vi "save_to_disk.vi"(1 "character string":string, 2 "Array":dbl[][](array[numeric]), 3 "File identifier":string) -> (0 "path":path)   [LabVIEW 2013]
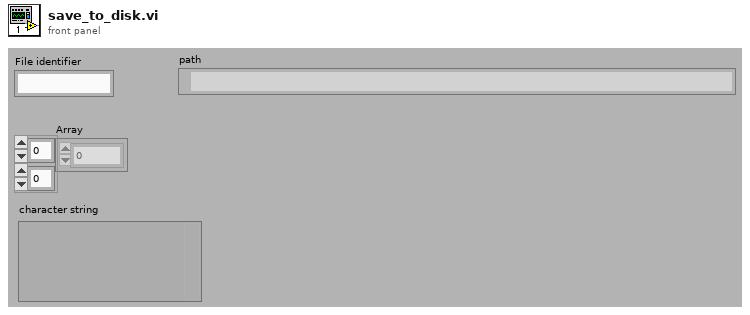
[diagram p1: front panel]
types:
  T1 = enum16{"open", "replace", "create", "open or create", "replace or create", "replace or create with confirmation"}
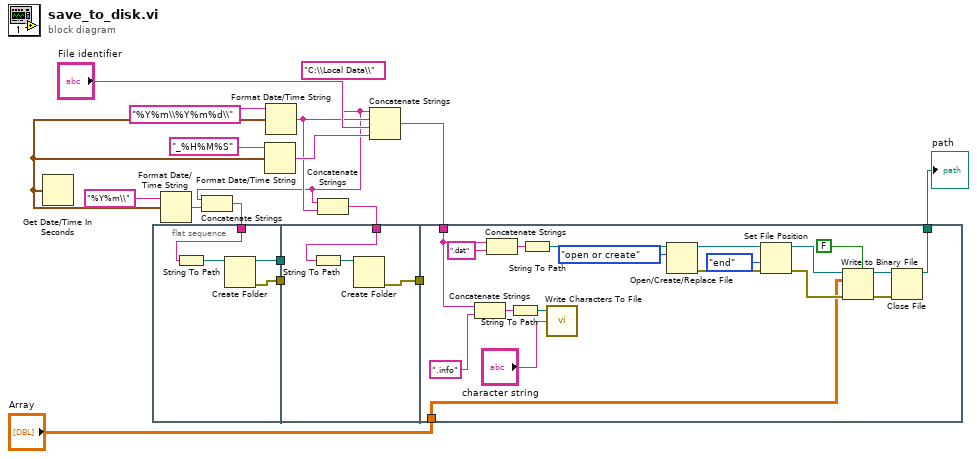
[diagram p0: block diagram]
diagram:
  w6 = "C:\\Local Data\\" ("string")
  n1 = Get Date/Time In Seconds() -> (seconds since 1Jan1904=w11:timestamp)
  n2 = flat-sequence {
    tunnel: [w21] -> w17
    tunnel: w4 -> [w20]
    tunnel: [w18] -> w1
    tunnel: w17 -> [_]
    tunnel: [w24] -> w16
    tunnel: w5 -> [w22]
    tunnel: w1 -> [_]
    tunnel: "Array" -> [w26]
    tunnel: w16 -> [_]
    tunnel: w3 -> [w40]
    tunnel: [w25] -> w2
    frame #0 {
      n3 = String To Path(string=w20) -> (path=w19:path)
      n4 = Create Folder(path (use dialog)=w19) -> (created path=w18:path, error out=w21:errorcluster)  [unwired: 2 in, 1 out]
    }
    frame #1 {
      n5 = String To Path(string=w22) -> (path=w23:path)
      n6 = Create Folder(path (use dialog)=w23) -> (error out=w24:errorcluster)  [unwired: 2 in, 2 out]
    }
    frame #2 {
      n7 = Concatenate Strings(w40, ".info" ("string")) -> (w38:string)
      n8 = Concatenate Strings(w40, ".dat" ("string")) -> (w43:string)
      n9 = String To Path(string=w38) -> (path=w39:path)
      n10 = String To Path(string=w43) -> (path=w28:path)
      n11 = call <vilib>:"Write Characters To File.vi"("character string"="character string", "file path (dialog if empty)"=w39) -> ()  [unwired: 3 in, 1 out]
      n12 = Open/Create/Replace File(file path (use dialog)=w28, operation (0:open)=T1."open or create") -> (refnum out=w35:refnum<file>, error out=w30:errorcluster)  [unwired: 4 in, 1 out]
      n13 = Set File Position(refnum=w35, from (0:start)=enum16{"start", "end", "current"}."end", error in=w30) -> (refnum out=w34:refnum<file>, error out=w31:errorcluster)  [unwired: 1 in]
      n14 = Write to Binary File(file (use dialog)=w34, data=w26, error in=w31, 5:FALSE ("prepend array or string size? (T)")) -> (refnum out=w32:refnum<file>, error out=w33:errorcluster)  [unwired: 2 in, 1 out]
      n15 = Close File(refnum=w32, error in=w33) -> (path=w25:path)  [unwired: 1 out]
    }
  }
  n16 = Format Date/Time String(time format string (%c)="%Y%m\\", seconds (now)=w11) -> (date/time string=w10:string)  [unwired: 1 in]
  n17 = Concatenate Strings(w6, w10) -> (w4:string)
  n18 = Format Date/Time String(time format string (%c)="_%H%M%S", seconds (now)=w11) -> (date/time string=w13:string)  [unwired: 1 in]
  n19 = Format Date/Time String(time format string (%c)="%Y%m\\%Y%m%d\\", seconds (now)=w11) -> (date/time string=w9:string)  [unwired: 1 in]
  n20 = Concatenate Strings(w6, w9) -> (w5:string)
  n21 = Concatenate Strings(w6, w9, "File identifier", w13) -> (w3:string)
  "path" <- w2
